vi "Reset Metodo.vi"(8 "error in (no error)":errorcluster, 11 "Keysight in":refnum<class "Edu-1200.lvclass">) -> (0 "error out":errorcluster, 3 "Keysight out":refnum<class "Edu-1200.lvclass">)   [LabVIEW 2020, in "Edu-1200.lvclass"]
uses:
  Edu-1200.lvclass
  Edu-1200.lvclass/Edu-1200.ctl
  <instrlib>/Agilent 2000 3000 X-Series/Agilent 2000 3000 X-Series.lvlib
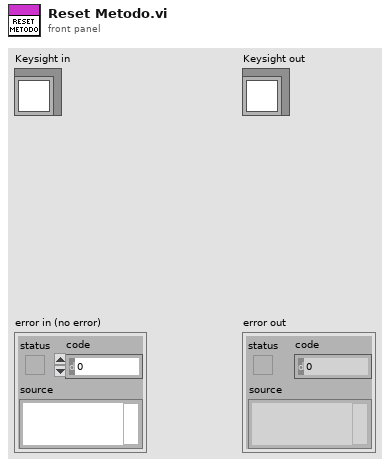
[diagram p1: front panel]
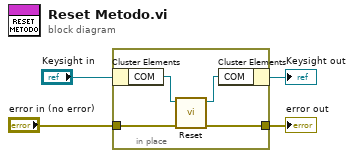
[diagram p0: block diagram]
diagram:
  n1 = in-place {
    in-place-border: [w6] -> w2
    in-place-border: "error in (no error)" -> [w5]
    n2 = in-place-cluster #1("Keysight in") -> ("COM"=w8:refnum<visa-resource-name>)
    n3 = call <instrlib>:"Reset.vi"("error in (no error)"=w5, "VISA resource name"=w8) -> ("error out"=w6:errorcluster, "VISA resource name out"=w7:refnum<visa-resource-name>)  [unwired: 8 in]
    n4 = in-place-cluster #1("COM"=w7) -> (→"Keysight out":refnum<class "Edu-1200.lvclass">)
  }
  "error out" <- w2
